vi "RT_Control_Adrian_MicrophonesWithAngle.vi"(10 "rt fifo":refnum<k33>, 11 "Parameters":T1={"N_chan"=0, "Input Rate (Hz)"=0.0, "Acq Time (s)"=0.0, "NumOfWarmupIters"=0, "Size fifo"=0, "Period NCL (ms)"=0, "Timeout fifo Read"=0, "Size Sent Array"=0, "Output offsets"=[], "Input offsets"=[0.0, 0.0, 0.0, 0.0, 0.0, 0.0, 0.0, 0.0]}) -> (0 "error out":errorcluster, 2 "Delayed Cycles":dbl)   [LabVIEW 2021]
uses:
  parametersRT.ctl
  <vilib>/DAQmx/write.llb/DAQmx Write (Analog 1D DBL NChan 1Samp).vi
  <vilib>/DAQmx/read.llb/DAQmx Read (Analog 1D DBL NChan 1Samp).vi
  <vilib>/DAQmx/read.llb/DAQmx Read (Digital 2D U32 NChan NSamp).vi
  <vilib>/Analysis/baseanly.llb/Mean (DBL).vi
  <vilib>/DAQmx/configure/timing.llb/DAQmx Timing (Sample Clock).vi
  <vilib>/DAQmx/miscellaneous.llb/DAQmx Fill In Error Info.vi
  <resource>/objmgr/daqmx.rc
  <vilib>/Analysis/NI_AALBase.lvlib
panel:
  out "data 2":u32[][](array[numeric])
  out "Encoder Raw Outputs":dbl[][](array[numeric])
  out "Encoder Mean Outputs":dbl[](array[numeric])
  in  "Zero Angle":dbl[](array[numeric])=[-16.79, 2.64, -15.0, 3.7]
  out "data":dbl[](array[numeric]) format="%0.2f"
  out "Numeric":i32
  out "output array":dbl[](array[numeric])
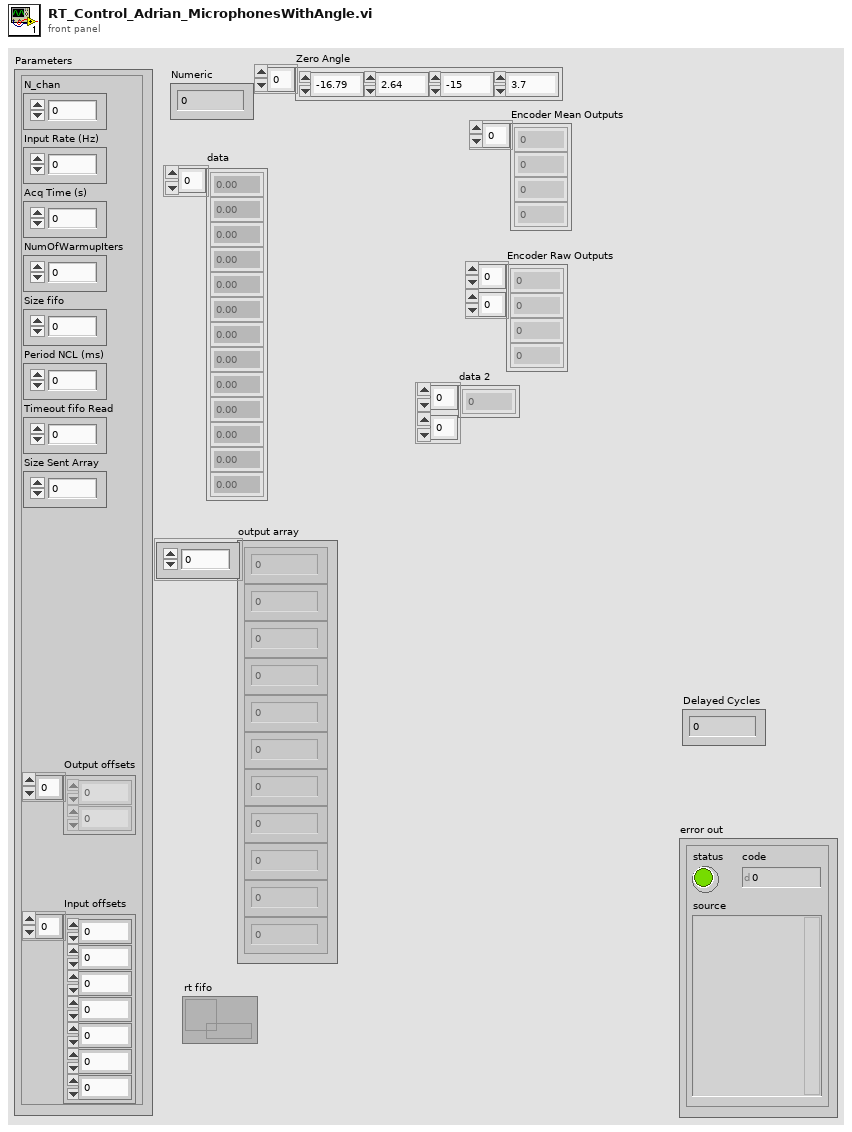
[diagram p1: front panel]
types:
  T1 = typedef "parametersRT.ctl" = cluster{"N_chan":u32, "Input Rate (Hz)":dbl, "Acq Time (s)":dbl, "NumOfWarmupIters":u32, "Size fifo":u32, "Period NCL (ms)":i64, "Timeout fifo Read":i32, "Size Sent Array":i32, "Output offsets":dbl[], "Input offsets":dbl[]}
  T2 = cluster{"Csn task out":refnum<k21>, "CLK task out":refnum<k21>, "D0 task out":refnum<k21>}
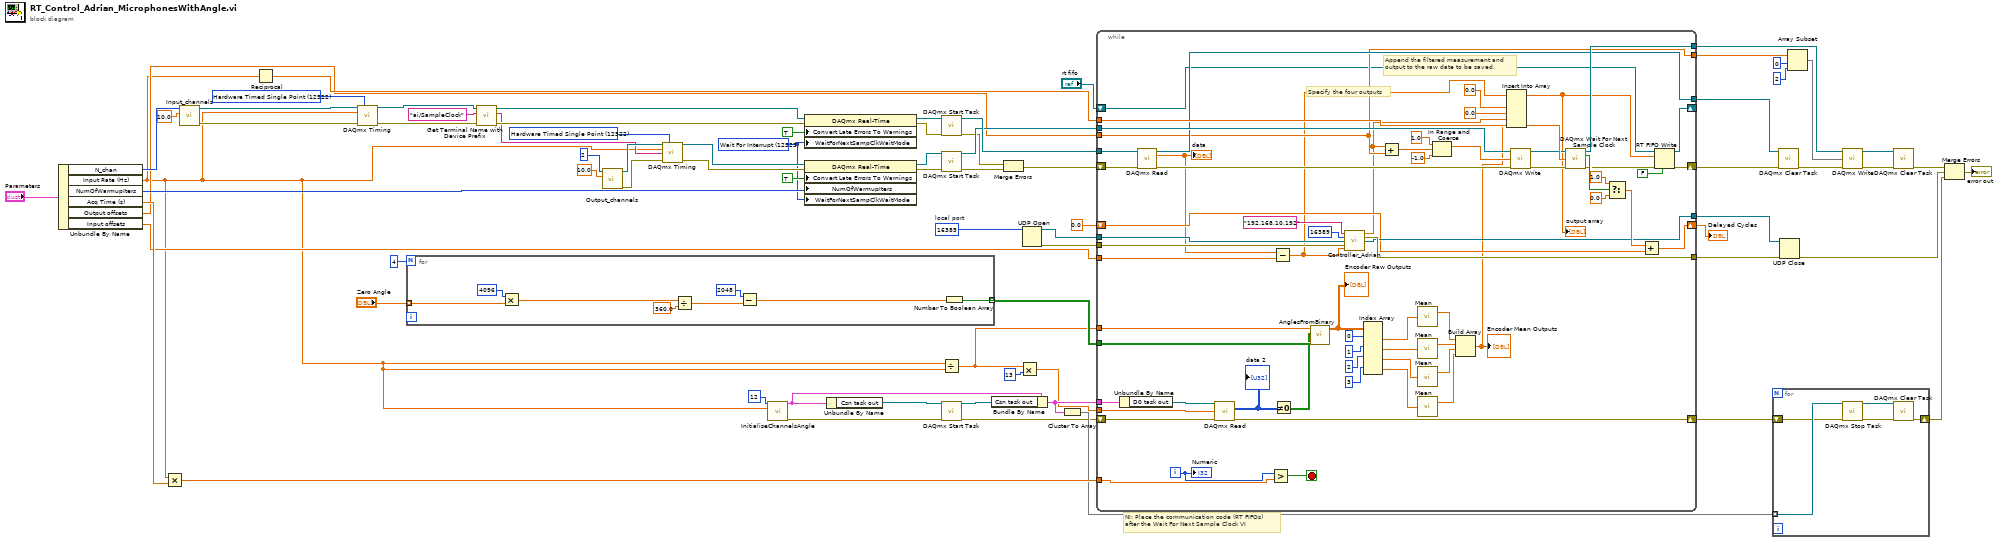
[diagram p0: block diagram]
diagram:
  w33 = u16 16385  # local port
  w40 = 12522 items=["Finite Samples"=10178, "Continuous Samples"=10123, "Hardware Timed Single Point"=12522] ("sample mode")
  w48 = 12523 items=["Wait For Interrupt"=12523, "Poll"=12524, "Yield"=12525] ("WaitForNextSampClkWaitMode")
  w74 = 12522 items=["Finite Samples"=10178, "Continuous Samples"=10123, "Hardware Timed Single Point"=12522] ("sample mode")
  # "NI: Place the communication code (RT FIFOs) \nafter the Wait For Next Sample Clock VI"
  n1 = Unbundle By Name("Parameters") -> ("N_chan"=w59:u32, "Input Rate (Hz)"=w1:dbl, "NumOfWarmupIters"=w60:u32, "Acq Time (s)"=w67:dbl, "Output offsets"=w58:dbl[], "Input offsets"=w49:dbl[])
  n2 = Multiply(x=w1, y=w67) -> (x*y=w27:dbl)
  n3 = call "Input_channels.vi"("Range"=10.0, "nchan"=w59) -> ("error out"=w42:errorcluster, "Refnum out"=w41:refnum<k21>)  [unwired: 8 in]
  n4 = Reciprocal(x=w1) -> (1/x=w73:dbl)
  n5 = call-poly <vilib>:"DAQmx Timing.vi"("task/channels in"=w41, "sample mode"=w40, "rate"=w1, "error in"=w42) -> ("task out"=w21:refnum<k21>, "error out"=w23:errorcluster)  [unwired: 10 in]
  n6 = for {
    N: 4 -> [_]
    tunnel: [w79] -> w5 mode=indexing
    tunnel: "Zero Angle" -> [w82] mode=indexing
    n7 = Multiply(x=4096, y=w82) -> (x*y=w83:dbl)
    n8 = Divide(x=w83, y=360.0) -> (x/y=w77:dbl)
    n9 = Subtract(x=2048, y=w77) -> (x-y=w76:dbl)
    n10 = Number To Boolean Array(number=w76) -> (Boolean array=w79:bool[])
  }
  n11 = call "Get Terminal Name with Device Prefix.vi"("error in (no error)"=w23, "Local Terminal Name"="ai/SampleClock", "task/channels in"=w21) -> ("error out"=w22:errorcluster, "Terminal Name with Device Prefix"=w19:tag, "task out"=w20:refnum<k21>)  [unwired: 6 in]
  n12 = call "Output_channels.vi"("Range"=10.0 ("Maximum Value"), "nchan"=2) -> ("error out"=w64:errorcluster, "Refnum out"=w63:refnum<k21>)  [unwired: 8 in]
  n13 = call-poly <vilib>:"DAQmx Timing.vi"("task/channels in"=w63, "sample mode"=w74, "rate"=w1, "source"=w19, "error in"=w64) -> ("task out"=w72:refnum<k21>, "error out"=w71:errorcluster)  [unwired: 9 in]
  n14 = call "InitialiseChannelsAngle.vi"("Number of data bits"=12, "Fs"=w1) -> ("output cluster"=w10:T2, "error out"=w11:errorcluster)  [unwired: 12 in]
  n15 = property class="DAQmx Real-Time"(reference=w20, error in=w22, "Convert Late Errors To Warnings"=TRUE, "WaitForNextSampClkWaitMode"=w48) -> (reference out=w37:refnum<k21>, error out=w36:errorcluster)
  n16 = property class="DAQmx Real-Time"(reference=w72, error in=w71, "Convert Late Errors To Warnings"=TRUE, "NumOfWarmupIters"=w60, "WaitForNextSampClkWaitMode"=w48) -> (reference out=w68:refnum<k21>, error out=w45:errorcluster)
  n17 = Unbundle By Name(w10) -> ("Csn task out"=w15:refnum<k21>)
  n18 = call <vilib>:"DAQmx Start Task.vi"("task/channels in"=w37, "error in"=w36) -> ("task out"=w66:refnum<k21>, "error out"=w35:errorcluster)  [unwired: 12 in]
  n19 = call <vilib>:"DAQmx Start Task.vi"("task/channels in"=w68, "error in"=w45) -> ("task out"=w65:refnum<k21>, "error out"=w44:errorcluster)  [unwired: 12 in]
  n20 = Divide(x=w1, y=w1) -> (x/y=w4:dbl)
  n21 = call <vilib>:"DAQmx Start Task.vi"("task/channels in"=w15, "error in"=w11) -> ("task out"=w14:refnum<k21>, "error out"=w6:errorcluster)  [unwired: 12 in]
  n22 = Bundle By Name(cluster=w10, "Csn task out"=w14) -> (w3:T2)
  n23 = Merge Errors(w35, w44) -> (w34:errorcluster)
  n24 = Multiply(x=w4, y=13) -> (x*y=w2:dbl)
  n25 = UDP Open(11:w33) -> (port=w31:refnum<k16>, 0:w32:errorcluster)  [unwired: 4 in, 1 out]
  n26 = Cluster To Array(cluster=w3) -> (array=w9:refnum<k21>[])
  n27 = while {
    shift-right: [w114] -> w43
    shift-left: w34 -> [w132]
    shift-right: [w144] -> w75
    shift-left: 0.0 ("f") -> [w119]
    tunnel: w73 -> [w142]
    tunnel: w27 -> [w140]
    tunnel: w65 -> [w138]
    tunnel: [w133] -> w69
    tunnel: w66 -> [w134]
    tunnel: [w136] -> w57
    tunnel: w58 -> [w127]
    tunnel: [w127] -> w52
    tunnel: w49 -> [w135]
    tunnel: w32 -> [w125]
    tunnel: w31 -> [w124]
    tunnel: [w123] -> w30
    tunnel: [w122] -> w29
    shift-right: [w110] -> _
    shift-left: "rt fifo" -> [w111]
    shift-right: [w91] -> w7
    shift-left: w6 -> [w90]
    tunnel: w5 -> [w89]
    tunnel: w4 -> [w88]
    tunnel: w3 -> [w87]
    tunnel: w2 -> [w86]
    i -> [w117]
    stop <- w141 stop-if-true
    # "Append the filtered measurement and \noutput to the raw date to be saved."
    # "Specify the four outputs"
    n28 = Unbundle By Name(w87) -> ("D0 task out"=w106:refnum<k21>)
    n29 = call-poly <vilib>:"DAQmx Read.vi"("task/channels in"=w134, "error in"=w132) -> ("task out"=w133:refnum<k21>, "data"=w116:dbl[], "error out"=w131:errorcluster)  [unwired: 11 in]
    "data" <- w116
    n30 = call-poly <vilib>:"DAQmx Read.vi"("task/channels in"=w106, "number of samples per channel"=w86, "error in"=w90) -> ("data"=w105:u32[][], "error out"=w91:errorcluster)  [unwired: 10 in, 1 out]
    "data 2" <- w105
    n31 = Greater?(x=w117, y=w140) -> (0:w141:bool)
    n32 = Subtract(x=w116, y=w135) -> (x-y=w118:dbl[])
    n33 = Not Equal To 0?(x=w105) -> (x != 0?=w85:bool[][])
    n34 = call "AnglesFromBinary.vi"("Binary Offset"=w89, "Array"=w85, "Buffer Length"=w88) -> ("Unwrapped Phase"=w104:dbl[][])  [unwired: 8 in]
    "Encoder Raw Outputs" <- w104
    n35 = call "Controller_Adrian.vi"("name 2"="192.168.10.192", "port or service name"=u16 16389, "connection ID"=w124, "error in (no error)"=w125, "x"=w118) -> ("*(type *) &x"=w109:dbl[], "error out"=w123:errorcluster, "connection ID out"=w122:refnum<k16>)  [unwired: 8 in]
    n36 = Index Array(array=w104, index (row) #1=0 ("index (row)"), index (row) #2=1 ("index (row)"), index (row) #3=2 ("index (row)"), index (row) #4=3 ("index (row)")) -> (element #1=w99:dbl[], element #2=w98:dbl[], element #3=w97:dbl[], element #4=w96:dbl[])  [unwired: 4 in]
    n37 = Add(x=w109, y=w127) -> (x+y=w129:dbl[])
    n38 = call-poly <vilib>:"Mean.vi"("X"=w99) -> ("mean"=w92:dbl)  [unwired: 1 out]
    n39 = call-poly <vilib>:"Mean.vi"("X"=w98) -> ("mean"=w93:dbl)  [unwired: 1 out]
    n40 = call-poly <vilib>:"Mean.vi"("X"=w97) -> ("mean"=w94:dbl)  [unwired: 1 out]
    n41 = call-poly <vilib>:"Mean.vi"("X"=w96) -> ("mean"=w95:dbl)  [unwired: 1 out]
    n42 = In Range and Coerce(upper limit=1.0, x=w129, lower limit=-1.0) -> (coerced(x)=w126:dbl[])  [unwired: 1 out]
    n43 = Build Array(w92, w93, w94, w95) -> (w84:dbl[])
    "Encoder Mean Outputs" <- w84
    n44 = Insert Into Array(array=w118, new element #1=0.0 ("new element/subarray"), new element #2=0.0 ("new element/subarray"), new element #3=w109, new element #4=w84) -> (w112:dbl[])  [unwired: 1 in]
    "output array" <- w112
    n45 = call-poly <vilib>:"DAQmx Write.vi"("task/channels in"=w138, "data"=w126, "error in"=w131) -> ("task out"=w137:refnum<k21>, "error out"=w139:errorcluster)  [unwired: 10 in, 1 out]
    n46 = call <vilib>:"DAQmx Wait For Next Sample Clock.vi"("task/channels in"=w137, "timeout (sec)"=w142, "error in"=w139) -> ("task out"=w136:refnum<k21>, "is late?"=w143:bool, "error out"=w113:errorcluster)  [unwired: 10 in]
    n47 = Select(t=1.0, s=w143, f=0.0) -> (s? t:f=w145:dbl)
    n48 = Add(x=w145, y=w119) -> (x+y=w144:dbl)
    n49 = RT FIFO Write(0:w111, 1:w112, 3:w113, 5:FALSE ("overwrite on timeout (T)")) -> (8:w110:refnum<k33>, 11:w114:errorcluster)  [unwired: 1 in, 2 out]
    "Numeric" <- w117
  }
  "Delayed Cycles" <- w75
  n50 = for {
    tunnel: w9 -> [w152] mode=indexing
    shift-right: [w148] -> w8
    shift-left: w7 -> [w150]
    n51 = call <vilib>:"DAQmx Stop Task.vi"("task/channels in"=w152, "error in"=w150) -> ("task out"=w151:refnum<k21>, "error out"=w149:errorcluster)  [unwired: 12 in]
    n52 = call <vilib>:"DAQmx Clear Task.vi"("task in"=w151, "error in"=w149) -> ("error out"=w148:errorcluster)  [unwired: 13 in]
  }
  n53 = call <vilib>:"DAQmx Clear Task.vi"("task in"=w69, "error in"=w43) -> ("error out"=w55:errorcluster)  [unwired: 13 in]
  n54 = UDP Close(connection ID=w29, 8:w30) -> (error out=w28:errorcluster)  [unwired: 1 out]
  n55 = Array Subset(array=w52, index=0, length=2) -> (w53:dbl[])
  n56 = call-poly <vilib>:"DAQmx Write.vi"("task/channels in"=w57, "data"=w53, "error in"=w55) -> ("task out"=w56:refnum<k21>, "error out"=w54:errorcluster)  [unwired: 10 in, 1 out]
  n57 = call <vilib>:"DAQmx Clear Task.vi"("task in"=w56, "error in"=w54) -> ("error out"=w47:errorcluster)  [unwired: 13 in]
  n58 = Merge Errors(w47, w28, w8) -> (→"error out":errorcluster)
